vi "DataTreeCtrl deleteData.vi"(8 "error in (no error)":errorcluster, 11 "DataTreeCtrl in":refnum<class "DataTreeCtrl.lvclass">) -> (0 "error out":errorcluster, 3 "DataTreeCtrl out":refnum<class "DataTreeCtrl.lvclass">)   [LabVIEW 2018, in "DataTreeCtrl.lvclass"]
uses:
  DataTreeCtrl.lvclass
  DataTreeCtrl.lvclass/DataTreeCtrl.ctl
  ctl/FMstateMachineEnum.ctl
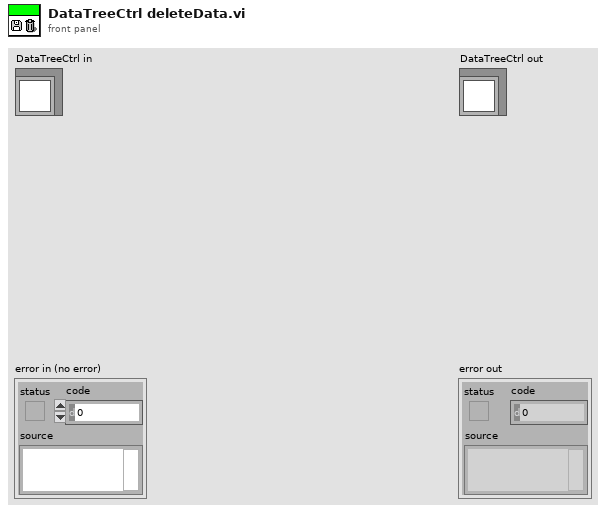
[diagram p1: front panel]
types:
  T1 = typedef "FMstateMachineEnum.ctl" = enum16{"none", "init", "openTDMS", "closeTDMS", "getDataList", "getDataInfo", "getTimeStamp", "getCurrPath", "getRemark", "overwriteRemark", "readData", "deleteData", "moveData"}
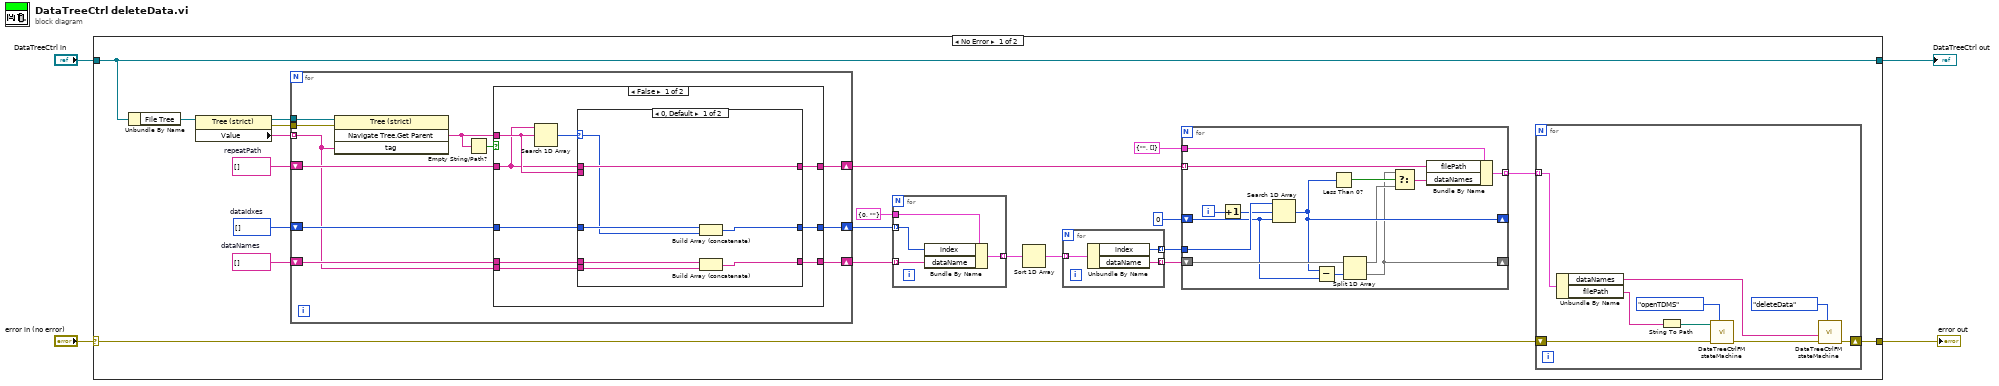
[diagram p0: block diagram]
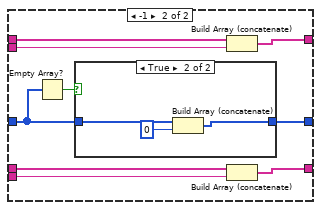
[diagram p2: hidden frame]
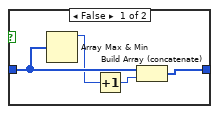
[diagram p3: hidden frame]
diagram:
  n1 = case shown="No Error" "error in (no error)" {
    selector: "error in (no error)" -> [w6 w103]
    tunnel: [w5 w103] -> w3
    tunnel: [w25 w102] -> w1
    tunnel: "DataTreeCtrl in" -> [w25 w102]
    frame No Error {
      w18 = string[] []  # dataNames
      w19 = i32[] []  # dataIdxes
      w20 = string[] []  # repeatPath
      n2 = Unbundle By Name(w25) -> ("File Tree"=w24:refnum<vi>)
      n3 = property class="Tree (strict)"(reference=w24) -> (reference out=w22:refnum<vi>, error out=w21:errorcluster, "Value"=w23:string[])  [unwired: 1 in]
      n4 = for {
        tunnel: w23 -> [w59] mode=indexing
        tunnel: w22 -> [w66]
        tunnel: w21 -> [w65]
        shift-right: [w56] -> w10
        shift-left: w20 -> [w62]
        shift-right: [w57] -> w9
        shift-left: w19 -> [w61]
        shift-right: [w58] -> w8
        shift-left: w18 -> [w60]
        n5 = invoke class="Tree (strict)" method="Navigate Tree.Get Parent"(reference=w66, error in=w65, "tag"=w59) -> ("Navigate Tree:Get Parent"=w64:string)  [unwired: 1 in, 3 out]
        n6 = Empty String/Path?(string/path=w64) -> (empty?=w63:bool)
        n7 = case shown="False" w63 {
          tunnel: w64 -> [w74 _]
          tunnel: w62 -> [w73 w100]
          tunnel: [w72 w100] -> w56
          tunnel: w61 -> [w71 w101]
          tunnel: w60 -> [w70 w99]
          tunnel: w59 -> [w69 _]
          tunnel: [w68 w99] -> w58
          tunnel: [w67 w101] -> w57
          frame False {
            n8 = Search 1D Array(1D array=w73, element=w74) -> (index of element=w75:i32)  [unwired: 1 in]
            n9 = case shown="0, Default" w75 {
              selector: w75 -> [w77 _]
              tunnel: w74 -> [_ w89]
              tunnel: w73 -> [w82 w91]
              tunnel: [w82 w90] -> w72
              tunnel: w71 -> [w78 w84]
              tunnel: w70 -> [w81 w88]
              tunnel: w69 -> [w80 w87]
              tunnel: [w79 w86] -> w68
              tunnel: [w76 w83] -> w67
              frame 0, Default {
                n10 = Build Array (concatenate)(w78, w77) -> (w76:i32[])
                n11 = Build Array (concatenate)(w81, w80) -> (w79:string[])
              }
              frame -1 {
                n12 = Empty Array?(array=w84) -> (empty?=w85:bool)
                n13 = case shown="True" w85 {
                  tunnel: w84 -> [w95 w98]
                  tunnel: [w94 w96] -> w83
                  frame False {
                    n14 = Array Max & Min(array=w95) -> (max value=w93:i32)  [unwired: 3 out]
                    n15 = Increment(x=w93) -> (x+1=w92:i32)
                    n16 = Build Array (concatenate)(w95, w92) -> (w94:i32[])
                  }
                  frame True {
                    n17 = Build Array (concatenate)(w98, 0) -> (w96:i32[])
                  }
                }
                n18 = Build Array (concatenate)(w91, w89) -> (w90:string[])
                n19 = Build Array (concatenate)(w88, w87) -> (w86:string[])
              }
            }
          }
          frame True {
          }
        }
      }
      n20 = for {
        tunnel: w9 -> [w52] mode=indexing
        tunnel: w8 -> [w54] mode=indexing
        tunnel: cluster{"index":i32, "dataName":string} {"index"=0, "dataName"=""} -> [w55]
        tunnel: [w53] -> w16 mode=indexing
        n21 = Bundle By Name(cluster=w55, "index"=w52, "dataName"=w54) -> (w53:cluster{"index":i32, "dataName":string})
      }
      n22 = Sort 1D Array(array=w16) -> (sorted array=w15:cluster{"index":i32, "dataName":string}[])
      n23 = for {
        tunnel: w15 -> [w51] mode=indexing
        tunnel: [w50] -> w14 mode=indexing
        tunnel: [w49] -> w13 mode=indexing
        n24 = Unbundle By Name(w51) -> ("index"=w50:i32, "dataName"=w49:string)
      }
      n25 = for {
        tunnel: w10 -> [w39] mode=indexing
        tunnel: w14 -> [w47]
        shift-right: [w42] -> _
        shift-left: 0 ("index of element") -> [w44]
        tunnel: cluster{"filePath":string, "dataNames":string[]} {"filePath"="", "dataNames"=[]} -> [w37]
        tunnel: [w36] -> w7 mode=indexing
        shift-right: [w35] -> _
        shift-left: w13 -> [w45]
        i -> [w48]
        n26 = Increment(x=w48) -> (x+1=w46:i32)
        n27 = Search 1D Array(1D array=w47, element=w46, start index (0)=w44) -> (index of element=w42:i32)
        n28 = Subtract(x=w42, y=w44) -> (x-y=w43:i32)
        n29 = Less Than 0?(x=w42) -> (x < 0?=w41:bool)
        n30 = Split 1D Array(array=w45, index=w43) -> (first subarray=w40:string[], second subarray=w35:string[])
        n31 = Select(t=w35, s=w41, f=w40) -> (s? t:f=w38:string[])
        n32 = Bundle By Name(cluster=w37, "filePath"=w39, "dataNames"=w38) -> (w36:cluster{"filePath":string, "dataNames":string[]})
      }
      n33 = for {
        tunnel: w7 -> [w29] mode=indexing
        shift-right: [w26] -> w5
        shift-left: w6 -> [w33]
        n34 = Unbundle By Name(w29) -> ("dataNames"=w27:string[], "filePath"=w32:string)
        n35 = String To Path(string=w32) -> (path=w31:path)
        n36 = call "DataTreeCtrlFM stateMachine.vi"("Func"=FMstateMachineEnum."openTDMS", "error in (no error)"=w33, "tdmsFilePath in"=w31) -> ("error out"=w28:errorcluster)  [unwired: 3 in, 5 out]
        n37 = call "DataTreeCtrlFM stateMachine.vi"("Func"=FMstateMachineEnum."deleteData", "error in (no error)"=w28, "multiDatasName"=w27) -> ("error out"=w26:errorcluster)  [unwired: 3 in, 5 out]
      }
    }
    frame Error {
    }
  }
  "error out" <- w3
  "DataTreeCtrl out" <- w1
